vi "Write Trigger.vi"(8 "error in (no error)":errorcluster, 10 "Trigger":T1={"Slope"=0, "Level"=0, "Source"=0, "External Range"=2000, "External Coupling"=0, "External"=FALSE, "Disable"=FALSE, "External Impedance"=1} {"External Impedance" items=["50 Ohm", "HiZ"]; "External Coupling" items=["DC", "AC"]; "External Range" min=2000 max=10000 step=8000; "Slope" items=["Rising", "Falling"]; "Level" min=-100 max=100; "Source" min=0 max=64 step=1}, 11 "Initialize_card in":refnum<class "Control_card.lvclass">) -> (0 "error out":errorcluster, 3 "Initialize_card out":refnum<class "Control_card.lvclass">)   [LabVIEW 2015, in "Control_card.lvclass"]
uses:
  Control_card.lvclass
  Control_card.lvclass/Control_card.ctl
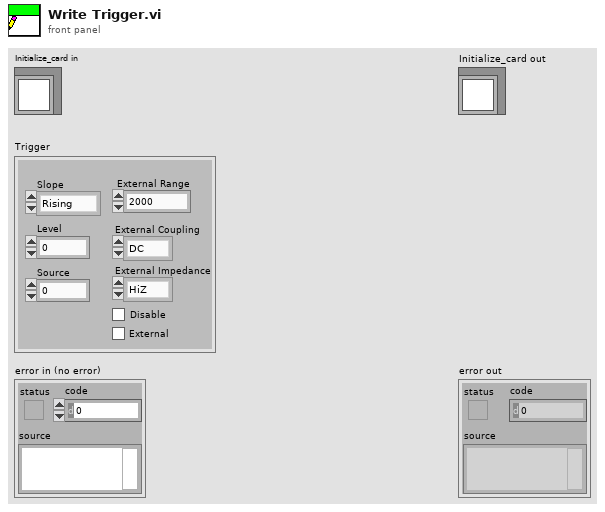
[diagram p1: front panel]
types:
  T1 = cluster{"Slope":u16, "Level":i32, "Source":i32, "External Range":u32, "External Coupling":u16, "External":bool, "Disable":bool, "External Impedance":u16}
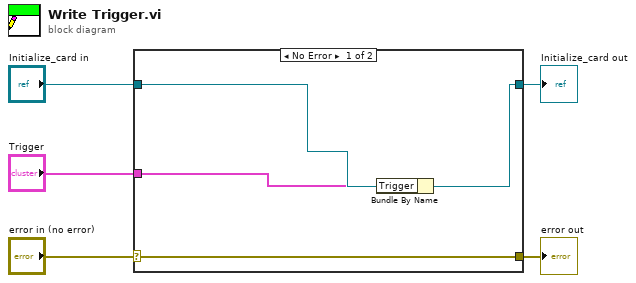
[diagram p0: block diagram]
diagram:
  n1 = case shown="No Error" "error in (no error)" {
    selector: "error in (no error)" -> [w9 w10]
    tunnel: [w9 w10] -> w4
    tunnel: [w7 w11] -> w2
    tunnel: "Initialize_card in" -> [w8 w11]
    tunnel: "Trigger" -> [w6 _]
    frame No Error {
      n2 = Bundle By Name(cluster=w8, "Trigger"=w6) -> (w7:refnum<class "Control_card.lvclass">)
    }
    frame Error {
    }
  }
  "error out" <- w4
  "Initialize_card out" <- w2
